vi "L5K Reader.vi"(8 "error in":errorcluster, 11 "L5K File Path":path) -> (0 "error out":errorcluster, 1 "Import Error":string, 2 "Tag Array":T1[](array[typedef]), 3 "L5K Information":T5)   [LabVIEW 2010, in "Ethernet IP Custom Device Custom Device.lvlib"]
uses:
  Ethernet IP Custom Device Custom Device.lvlib
  L5K Internal Data.ctl
  L5K Tag.ctl
  L5K Tag Name.ctl
  Result Source.ctl
  L5K Data Types.ctl
  ST Enum.ctl
panel:
  out "IP Address":string
  in  "Import Error - Array":string="\n%s - Reason: this tag is a multidimensional array. VeriStand EtherNet/IP add-on only support 1D array tags."
  in  "Import Error - Data Type":string="\n%s - Reason: the data type of this tag is not supported by the VeriStand EtherNet/IP add-on. Enter this tag manually with a generic datatype."
  in  "Import Error":string="VeriStand EtherNet/IP add-on did not import the following tags:\n"
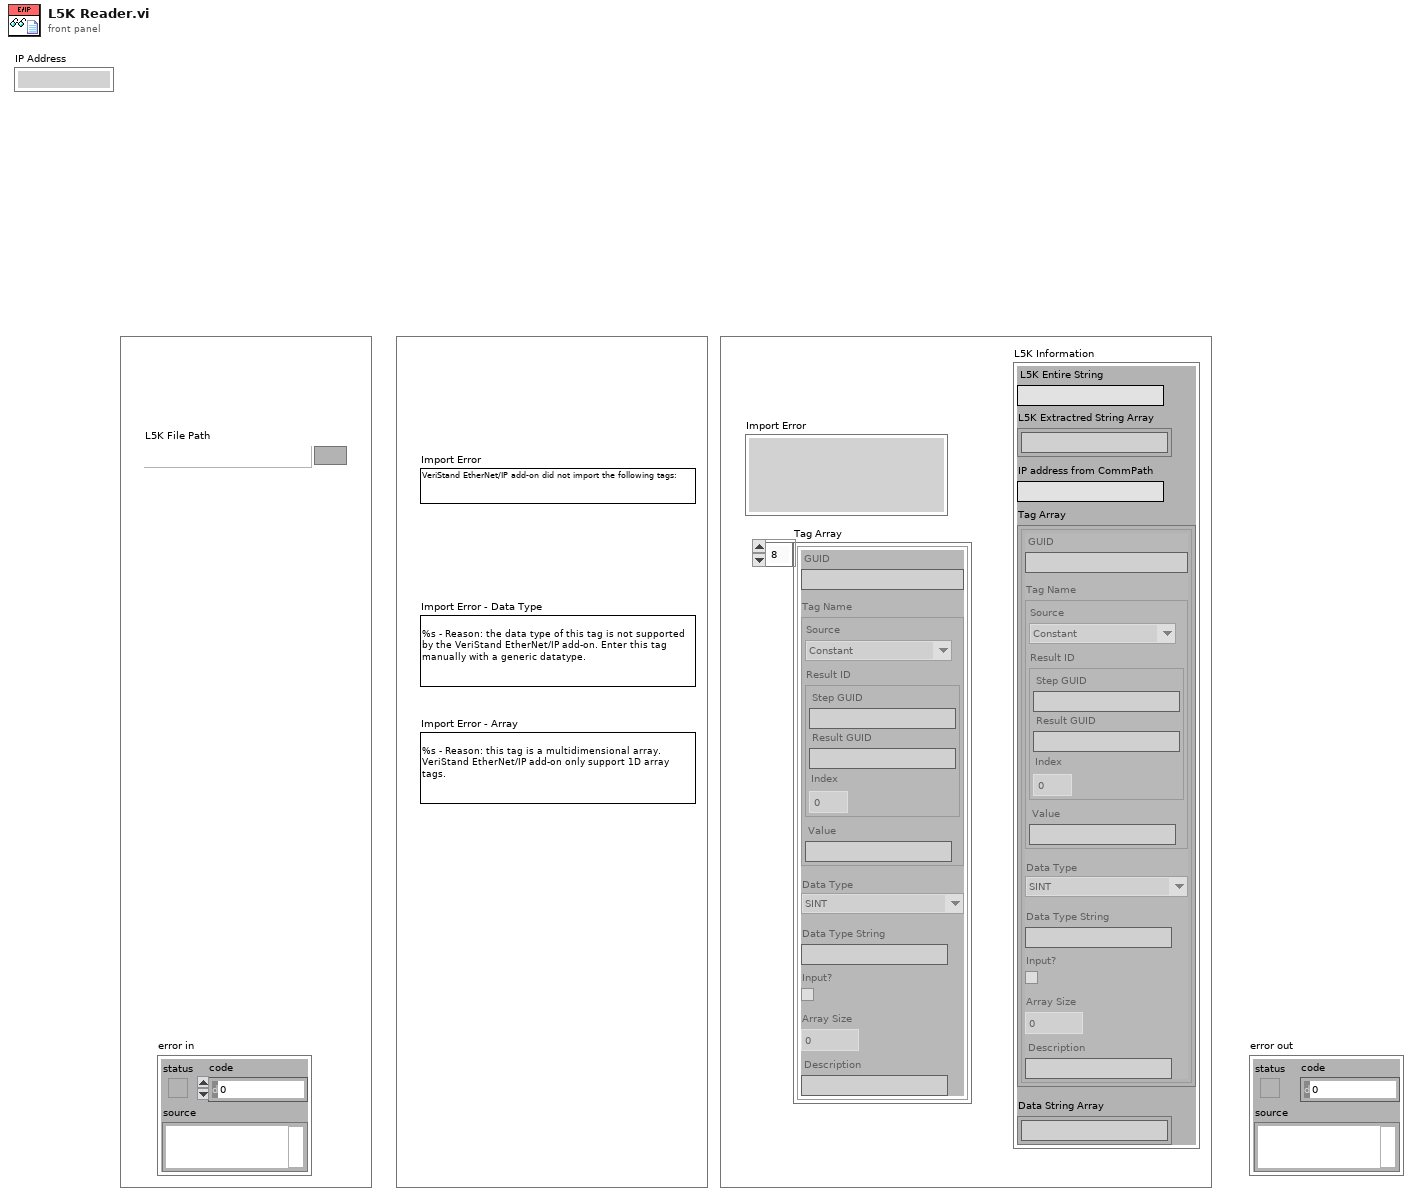
[diagram p1: front panel]
types:
  T1 = typedef "Ethernet IP Custom Device Custom Device.lvlib/L5K Tag.ctl" = cluster{"GUID":string, "Tag Name":T2, "Data Type":T4, "Data Type String":string, "Array Size":i32, "Description":string, "Input?":bool}
  T2 = typedef "Ethernet IP Custom Device Custom Device.lvlib/L5K Tag Name.ctl" = cluster{"Source":T3, "Result ID":cluster{"Step GUID":string, "Result GUID":string, "Index":dbl}, "Value":string}
  T3 = typedef "Ethernet IP Custom Device Custom Device.lvlib/Result Source.ctl" = enum16{"Constant", "Measure"}
  T4 = typedef "Ethernet IP Custom Device Custom Device.lvlib/L5K Data Types.ctl" = enum16{"SINT", "INT", "DINT", "REAL", "BOOL", "STRING"}
  T5 = typedef "Ethernet IP Custom Device Custom Device.lvlib/L5K Internal Data.ctl" = cluster{"L5K Entire String":string, "L5K Extractred String Array":string[], "IP address from CommPath":string, "Tag Array":T1[], "Data String Array":string[]}
  T6 = typedef "Ethernet IP Custom Device Custom Device.lvlib/ST Enum.ctl" = enum16{"Init", "Extract Strings", "Extract Tags", "Exit"}
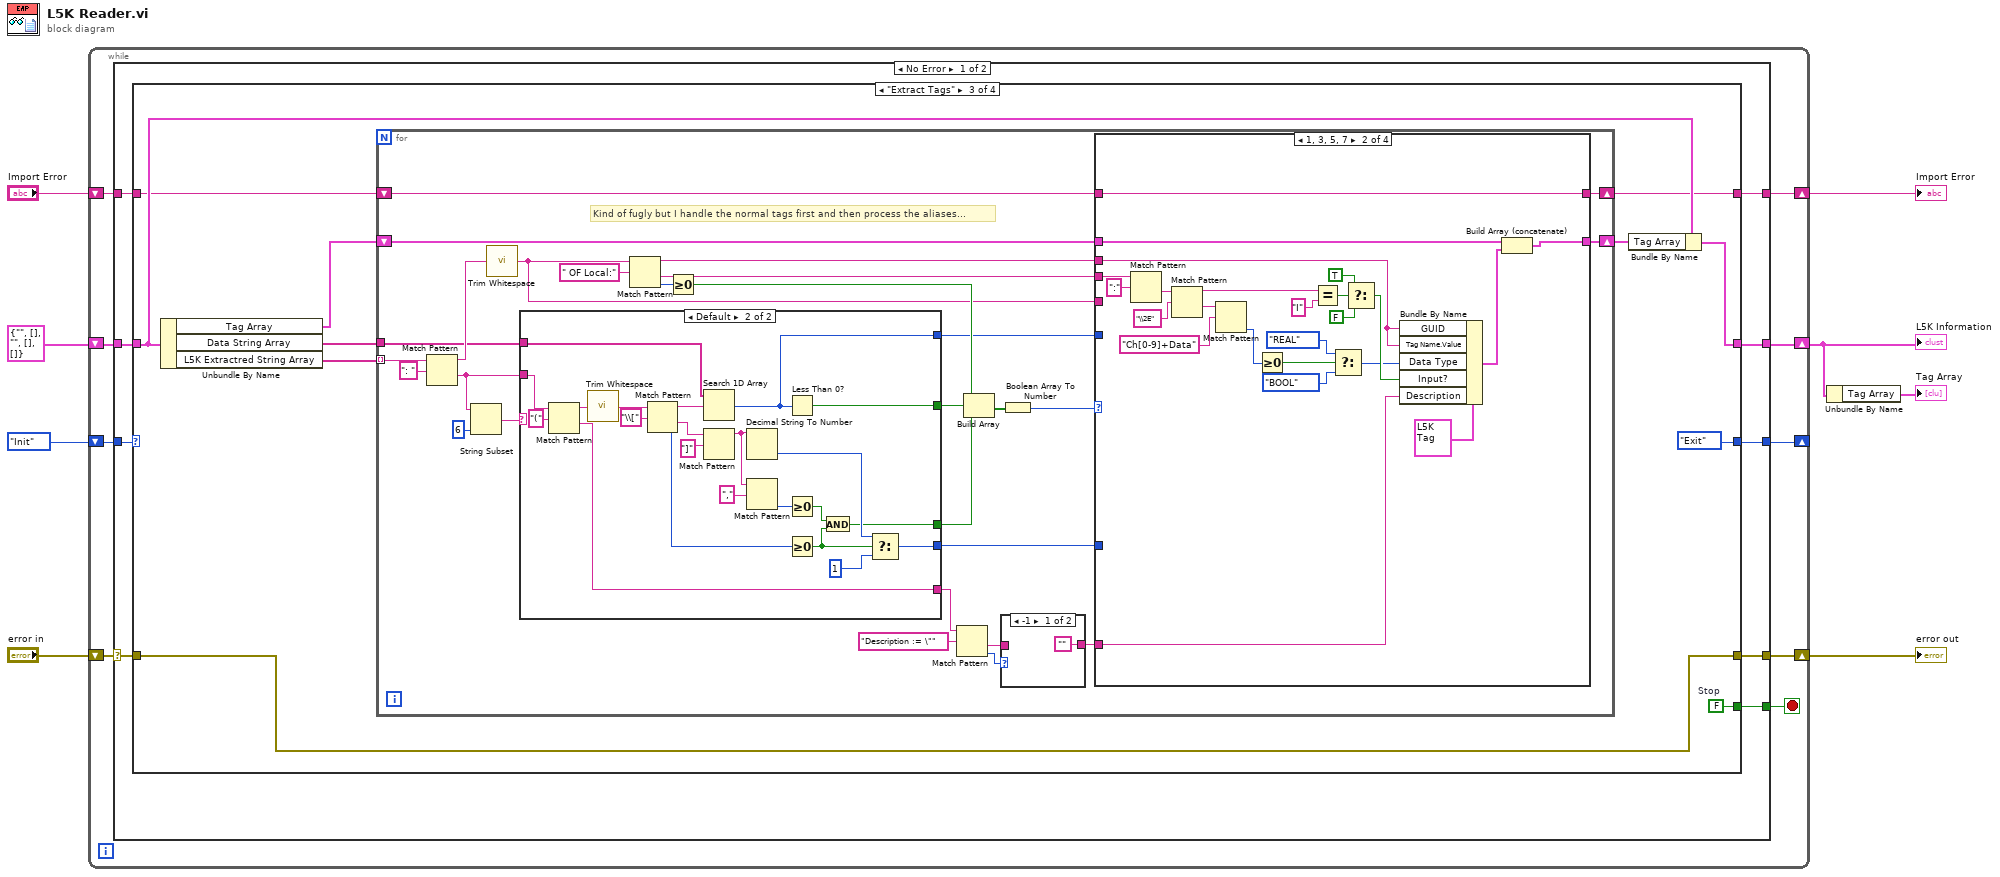
[diagram p0: block diagram]
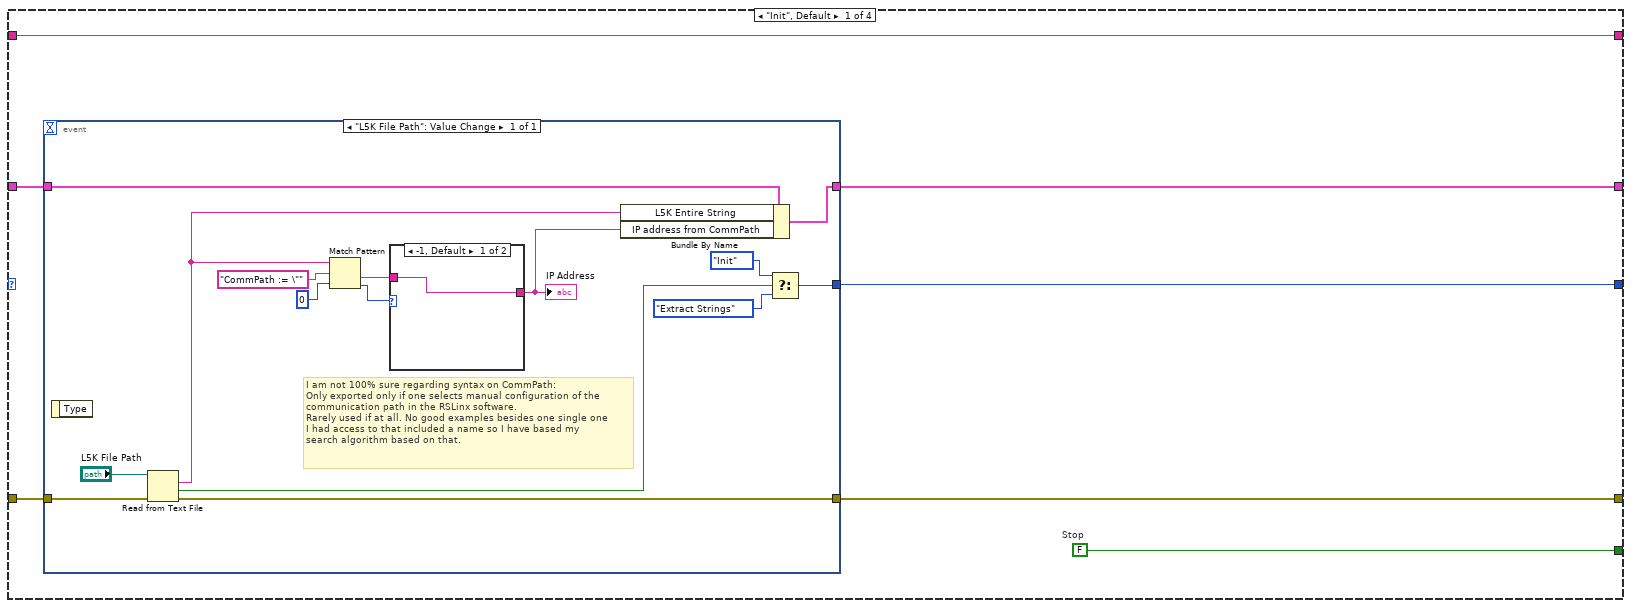
[diagram p2: hidden frame]
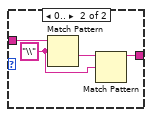
[diagram p3: hidden frame]
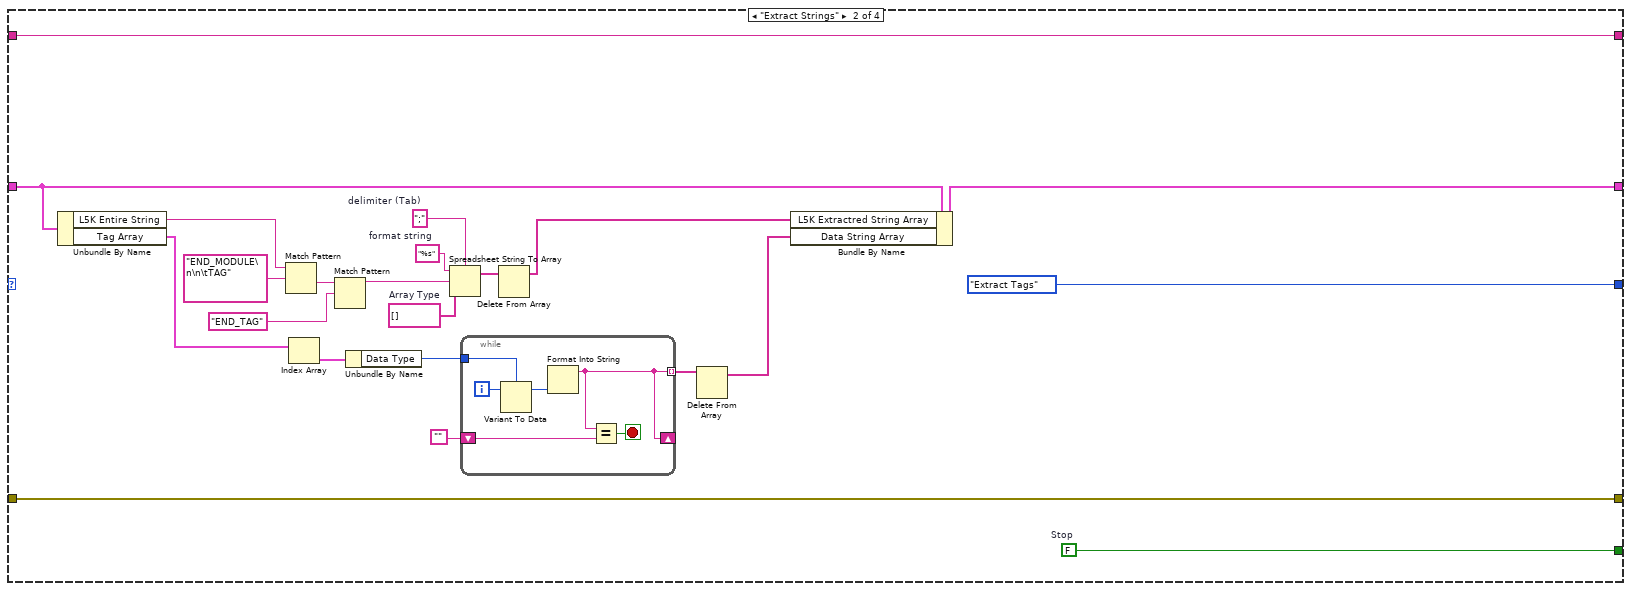
[diagram p4: hidden frame]
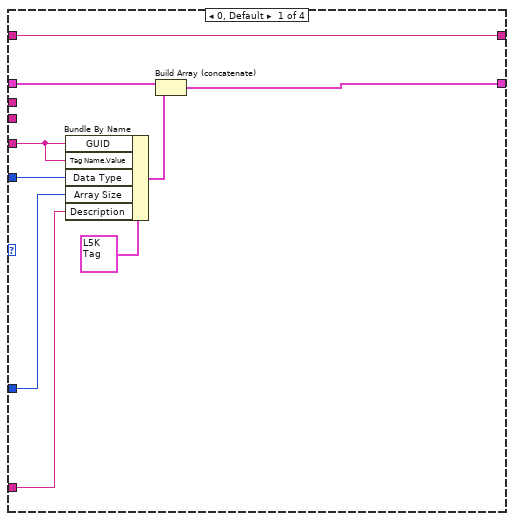
[diagram p5: hidden frame]
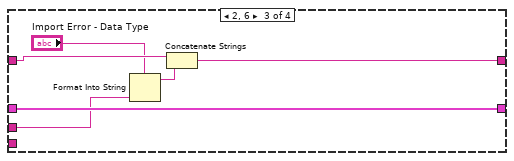
[diagram p6: hidden frame]
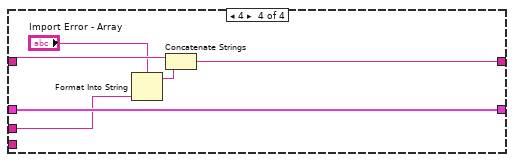
[diagram p7: hidden frame]
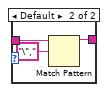
[diagram p8: hidden frame]
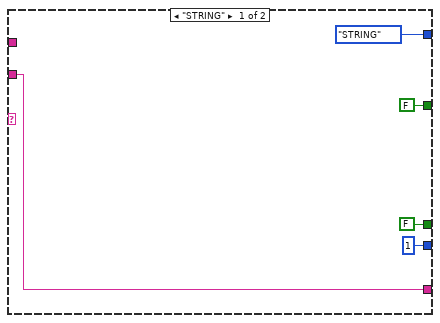
[diagram p9: hidden frame]
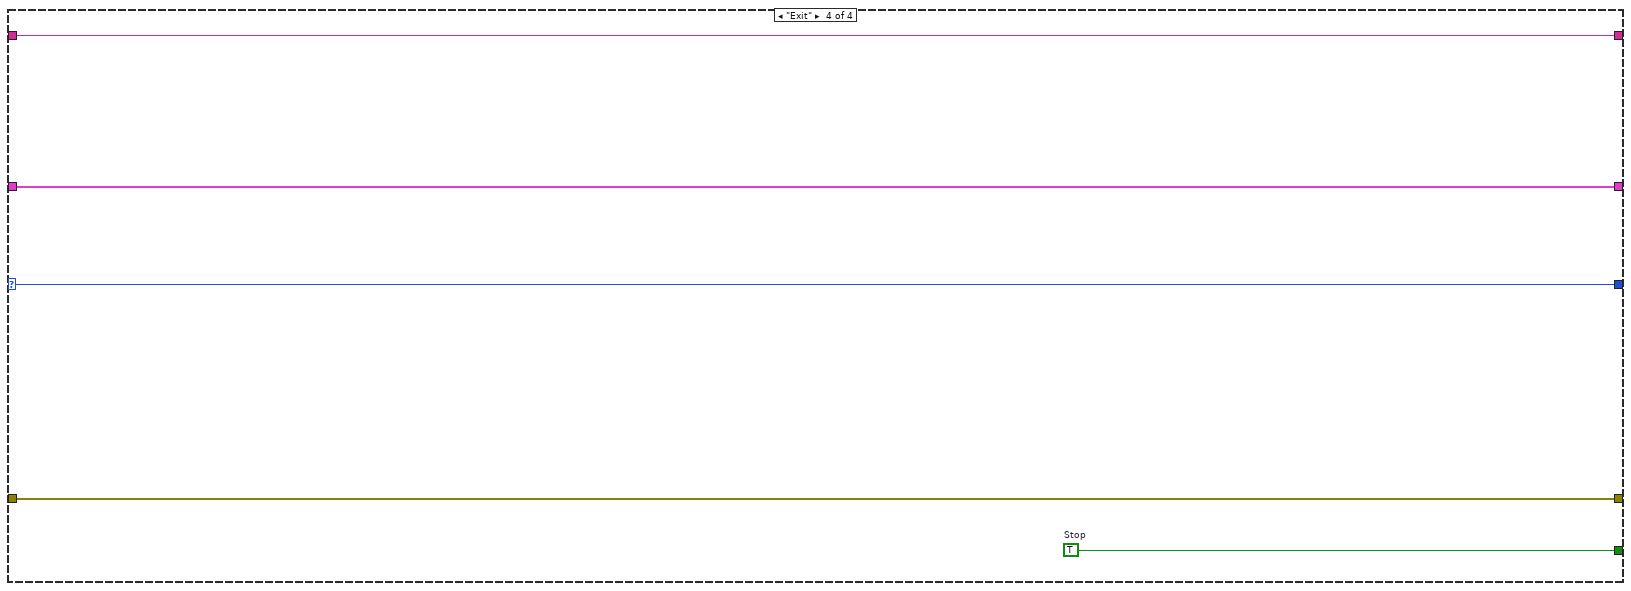
[diagram p10: hidden frame]
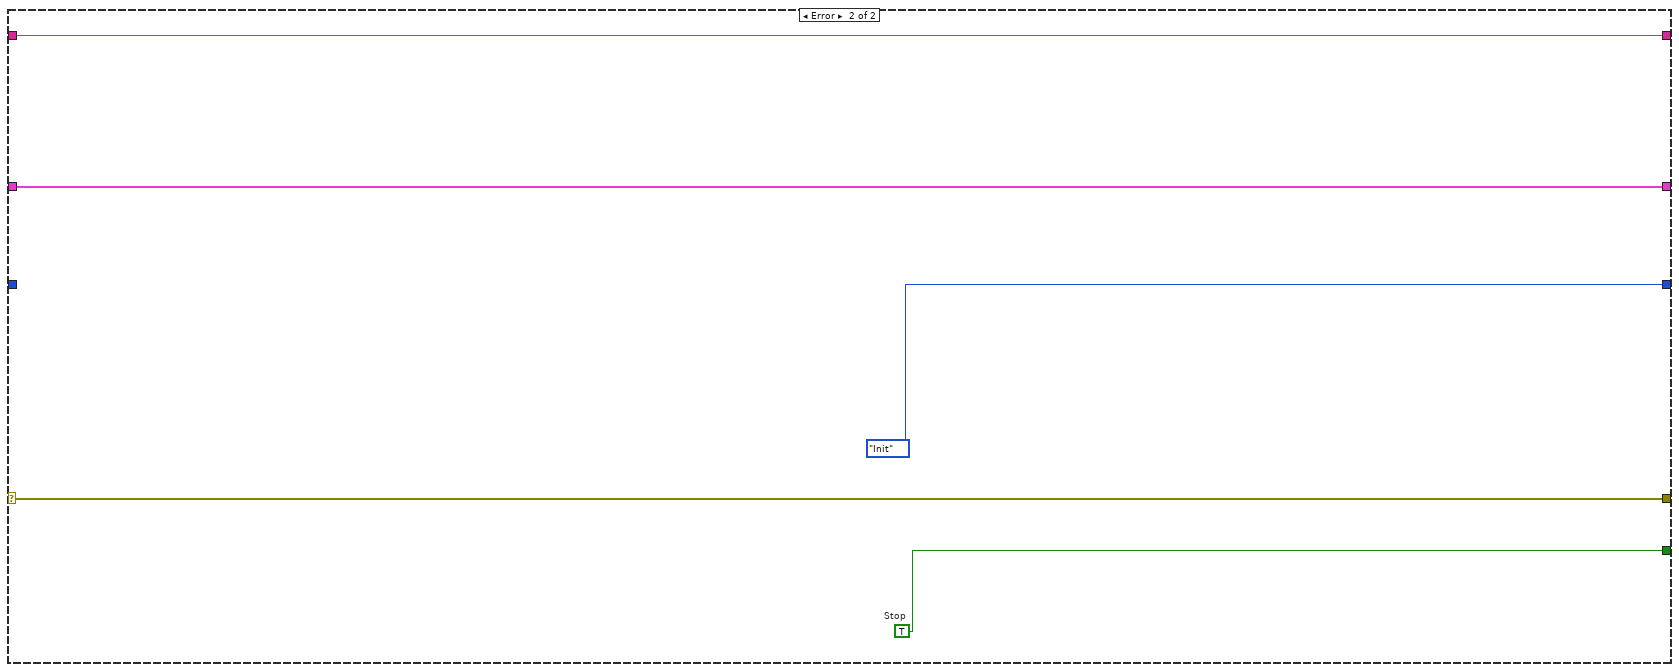
[diagram p11: hidden frame]
diagram:
  n1 = while {
    shift-right: [w15] -> _
    shift-left: ST_Enum."Init" ("Enum") -> [w17]
    shift-right: [w14] -> w5
    shift-left: "error in" -> [w11]
    shift-right: [w12] -> w2
    shift-left: T5 {"L5K Entire String"="", "L5K Extractred String Array"=[], "IP address from CommPath"="", "Tag Array"=[], "Data String Array"=[]} ("L5K Information") -> [w13]
    shift-right: [w9] -> w3
    shift-left: "Import Error" -> [w10]
    stop <- w16 stop-if-true
    n2 = case shown="No Error" w11 {
      selector: w11 -> [w20 w206]
      tunnel: w17 -> [w26 _]
      tunnel: [w25 w203] -> w16
      tunnel: [w24 ST_Enum."Init" ("Enum")] -> w15
      tunnel: [w23 w206] -> w14
      tunnel: w13 -> [w22 w205]
      tunnel: [w21 w205] -> w12
      tunnel: w10 -> [w19 w202]
      tunnel: [w18 w202] -> w9
      frame No Error {
        n3 = case shown="\"Extract Tags\"" w26 {
          selector: w26 -> [_ _ _ w200]
          tunnel: [w33 w62 w84 w201] -> w25
          tunnel: [w32 ST_Enum."Extract Tags" ("Enum") ST_Enum."Exit" ("Enum") w200] -> w24
          tunnel: w20 -> [w31 w63 w85 w199]
          tunnel: [w30 w63 w85 w199] -> w23
          tunnel: w22 -> [w29 w66 w89 w198]
          tunnel: [w28 w64 w87 w198] -> w21
          tunnel: w19 -> [w27 w54 w83 w197]
          tunnel: [w27 w54 w82 w197] -> w18
          frame "Init", Default {
            w33 = FALSE  # Stop
            n4 = event shown="[0] \"L5K File Path\": Value Change" {
              selector: _ -> [_]
              dyn-events: _ -> [_]
              timeout: _ -> [_]
              tunnel: [w44] -> w32
              tunnel: w31 -> [w43]
              tunnel: [w42] -> w30
              tunnel: w29 -> [w41]
              tunnel: [w40] -> w28
              event "L5K File Path": Value Change {
                # "I am not 100% sure regarding syntax on CommPath:\nOnly exported only if one selects manual configuration of the \ncommunication path in the RSLinx software.\nRarely used if at all. No good examples besides one single one\nI had access to that included a name so I have based my\nsearch algorithm based on that."
                n5 = event-data() -> ()  [unwired: 1 in, 1 out]
                n6 = Read from Text File(file (use dialog)="L5K File Path", error in=w43) -> (text=w36:string, cancelled=w47:bool, error out=w42:errorcluster)  [unwired: 2 in, 1 out]
                n7 = Match Pattern(string=w36, regular expression="CommPath := \"", offset (0)=0) -> (after substring=w38:string, offset past match=w37:i32)  [unwired: 2 out]
                n8 = case shown="-1, Default" w37 {
                  tunnel: w38 -> [w49 w53]
                  tunnel: [w49 w50] -> w35
                  frame -1, Default {
                  }
                  frame 0.. {
                    w51 = "\\" ("regular expression")
                    n9 = Match Pattern(string=w53, regular expression=w51) -> (after substring=w52:string)  [unwired: 1 in, 3 out]
                    n10 = Match Pattern(string=w52, regular expression=w51) -> (before substring=w50:string)  [unwired: 1 in, 3 out]
                  }
                }
                "IP Address" <- w35
                n11 = Bundle By Name(cluster=w41, "L5K Entire String"=w36, "IP address from CommPath"=w35) -> (w40:T5)
                n12 = Select(t=ST_Enum."Init" ("Enum"), s=w47, f=ST_Enum."Extract Strings" ("Enum")) -> (s? t:f=w44:T6)
              }
            }
          }
          frame "Extract Strings" {
            w62 = FALSE  # Stop
            w74 = string[] []  # Array Type
            w73 = ";"  # delimiter (Tab)
            w72 = "%s"  # format string
            n13 = Unbundle By Name(w66) -> ("L5K Entire String"=w67:string, "Tag Array"=w60:T1[])
            n14 = Match Pattern(string=w67, regular expression="END_MODULE\n\n\tTAG") -> (after substring=w69:string)  [unwired: 1 in, 3 out]
            n15 = Index Array(array=w60) -> (element=w59:T1)  [unwired: 1 in]
            n16 = Match Pattern(string=w69, regular expression="END_TAG") -> (before substring=w71:string)  [unwired: 1 in, 3 out]
            n17 = Unbundle By Name(w59) -> ("Data Type"=w57:T4)
            n18 = Spreadsheet String To Array(delimiter (Tab)=w73, format string=w72, spreadsheet string=w71, array type (2D Dbl)=w74) -> (array=w75:string[])
            n19 = while {
              shift-right: [w76] -> _
              shift-left: "" -> [w80]
              tunnel: w57 -> [w79]
              tunnel: [w76] -> w56 mode=indexing
              i -> [w78]
              stop <- w81 stop-if-true
              n20 = Variant To Data(Variant=w78, type=w79) -> (data=w77:T4)  [unwired: 1 in, 1 out]
              n21 = Format Into String(w77) -> (resulting string=w76:string)  [unwired: 3 in, 1 out]
              n22 = Equal?(x=w76, y=w80) -> (x = y?=w81:bool)
            }
            n23 = Delete From Array(array=w75) -> (array with subset deleted=w65:string[])  [unwired: 2 in, 1 out]
            n24 = Delete From Array(array=w56) -> (array with subset deleted=w55:string[])  [unwired: 2 in, 1 out]
            n25 = Bundle By Name(cluster=w66, "L5K Extractred String Array"=w65, "Data String Array"=w55) -> (w64:T5)
          }
          frame "Extract Tags" {
            w84 = FALSE  # Stop
            n26 = Unbundle By Name(w89) -> ("Tag Array"=w90:T1[], "Data String Array"=w91:string[], "L5K Extractred String Array"=w92:string[])
            n27 = for {
              tunnel: w92 -> [w117] mode=indexing
              tunnel: w91 -> [w114]
              shift-right: [w97] -> w88
              shift-left: w90 -> [w98]
              shift-right: [w95] -> w82
              shift-left: w83 -> [w94]
              # "Kind of fugly but I handle the normal tags first and then process the aliases..."
              n28 = Match Pattern(string=w117, regular expression=": ") -> (before substring=w119:string, after substring=w115:string)  [unwired: 1 in, 2 out]
              n29 = String Subset(string=w115, length (rest)=6 ("length (rest)")) -> (substring=w116:string)  [unwired: 1 in]
              n30 = call <vilib>:"Trim Whitespace.vi"("string"=w119) -> ("trimmed string"=w102:string)  [unwired: 1 in]
              n31 = case shown="Default" w116 {
                tunnel: w115 -> [w174 w182]
                tunnel: w114 -> [_ w180]
                tunnel: [w174 w179] -> w108
                tunnel: [FALSE w178] -> w106
                tunnel: [FALSE w177] -> w105
                tunnel: [L5K_Data_Types."STRING" ("Data Type") w176] -> w101
                tunnel: [1 ("t") w175] -> w100
                frame "STRING" {
                }
                frame Default {
                  n32 = Match Pattern(string=w182, regular expression="(") -> (before substring=w184:string, after substring=w179:string)  [unwired: 1 in, 2 out]
                  n33 = call <vilib>:"Trim Whitespace.vi"("string"=w184) -> ("trimmed string"=w185:string)  [unwired: 1 in]
                  n34 = Match Pattern(string=w185, regular expression="\\[") -> (before substring=w187:string, after substring=w188:string, offset past match=w192:i32)  [unwired: 1 in, 1 out]
                  n35 = Search 1D Array(1D array=w180, element=w187) -> (index of element=w176:i32)  [unwired: 1 in]
                  n36 = Match Pattern(string=w188, regular expression="]") -> (before substring=w191:string)  [unwired: 1 in, 3 out]
                  n37 = Decimal String To Number(string=w191) -> (number=w183:i32)  [unwired: 2 in, 1 out]
                  n38 = Match Pattern(string=w191, regular expression=",") -> (offset past match=w194:i32)  [unwired: 1 in, 3 out]
                  n39 = Less Than 0?(x=w176) -> (x < 0?=w177:bool)
                  n40 = Greater Or Equal To 0?(x=w194) -> (x >= 0?=w195:bool)
                  n41 = Greater Or Equal To 0?(x=w192) -> (x >= 0?=w196:bool)
                  n42 = And(x=w195, y=w196) -> (x .and. y?=w178:bool)
                  n43 = Select(t=w183, s=w196, f=1 ("t")) -> (s? t:f=w175:i32)
                }
              }
              n44 = Match Pattern(string=w102, regular expression=" OF Local:") -> (before substring=w96:string, after substring=w93:string, offset past match=w112:i32)  [unwired: 1 in, 1 out]
              n45 = Greater Or Equal To 0?(x=w112) -> (x >= 0?=w104:bool)
              n46 = Match Pattern(string=w108, regular expression="Description := \"") -> (after substring=w109:string, offset past match=w110:i32)  [unwired: 1 in, 2 out]
              n47 = Build Array(w104, w105, w106) -> (w107:bool[])
              n48 = case shown="-1" w110 {
                tunnel: ["" w168] -> w99
                tunnel: w109 -> [_ w167]
                frame -1 {
                }
                frame Default {
                  n49 = Match Pattern(string=w167, regular expression="\",") -> (before substring=w168:string)  [unwired: 1 in, 3 out]
                }
              }
              n50 = Boolean Array To Number(Boolean array=w107) -> (number=w103:u32)
              n51 = case shown="1, 3, 5, 7" w103 {
                tunnel: w102 -> [w128 _ _ _]
                tunnel: w101 -> [w127 _ _ _]
                tunnel: w100 -> [w126 _ _ _]
                tunnel: w99 -> [w125 w144 _ _]
                tunnel: w98 -> [w124 w143 w159 w165]
                tunnel: [w122 w141 w159 w165] -> w97
                tunnel: w96 -> [_ w146 w155 w161]
                tunnel: [w121 w142 w158 w164] -> w95
                tunnel: w94 -> [w121 w142 w156 w162]
                tunnel: w93 -> [_ w153 _ _]
                frame 0, Default {
                  n52 = Bundle By Name(cluster=T1 {"GUID"="", "Tag Name"={"Source"=enum."Constant", "Result ID"={"Step GUID"="", "Result GUID"="", "Index"=0.0}, "Value"=""}, "Data Type"=enum."SINT", "Data Type String"="", "Array Size"=0, "Description"="", "Input?"=FALSE} ("Tag"), "GUID"=w128, "Tag Name.Value"=w128, "Data Type"=w127, "Array Size"=w126, "Description"=w125) -> (w123:T1)
                  n53 = Build Array (concatenate)(w124, w123) -> (w122:T1[])
                }
                frame 1, 3, 5, 7 {
                  n54 = Match Pattern(string=w153, regular expression=":") -> (after substring=w140:string)  [unwired: 1 in, 3 out]
                  n55 = Match Pattern(string=w140, regular expression="\\2E") -> (before substring=w131:string, after substring=w139:string)  [unwired: 1 in, 2 out]
                  n56 = Match Pattern(string=w139, regular expression="Ch[0-9]+Data") -> (offset past match=w137:i32)  [unwired: 1 in, 3 out]
                  n57 = Greater Or Equal To 0?(x=w137) -> (x >= 0?=w136:bool)
                  n58 = Equal?(x=w131, y="I") -> (x = y?=w151:bool)
                  n59 = Select(t=L5K_Data_Types."REAL" ("Data Type"), s=w136, f=L5K_Data_Types."BOOL" ("Data Type")) -> (s? t:f=w135:T4)
                  n60 = Select(t=TRUE, s=w151, f=FALSE) -> (s? t:f=w145:bool)
                  n61 = Bundle By Name(cluster=T1 {"GUID"="", "Tag Name"={"Source"=enum."Constant", "Result ID"={"Step GUID"="", "Result GUID"="", "Index"=0.0}, "Value"=""}, "Data Type"=enum."SINT", "Data Type String"="", "Array Size"=0, "Description"="", "Input?"=FALSE} ("Tag"), "GUID"=w146, "Tag Name.Value"=w146, "Data Type"=w135, "Input?"=w145, "Description"=w144) -> (w147:T1)
                  n62 = Build Array (concatenate)(w143, w147) -> (w141:T1[])
                }
                frame 2, 6 {
                  n63 = Format Into String(format string="Import Error - Data Type", w155) -> (resulting string=w157:string)  [unwired: 2 in, 1 out]
                  n64 = Concatenate Strings(w156, w157) -> (w158:string)
                }
                frame 4 {
                  n65 = Format Into String(format string="Import Error - Array", w161) -> (resulting string=w163:string)  [unwired: 2 in, 1 out]
                  n66 = Concatenate Strings(w162, w163) -> (w164:string)
                }
              }
            }
            n67 = Bundle By Name(cluster=w89, "Tag Array"=w88) -> (w87:T5)
          }
          frame "Exit" {
            w201 = TRUE  # Stop
          }
        }
      }
      frame Error {
        w203 = TRUE  # Stop
      }
    }
  }
  "error out" <- w5
  "Import Error" <- w3
  "L5K Information" <- w2
  n68 = Unbundle By Name(w2) -> ("Tag Array"=→"Tag Array":T1[])
